vi "mtg reader - recolor folder list.vi"(6 "max index":i32, 9 "Row in":i32, 11 "table ref":refnum<vi>) -> (1 "Row out":i32, 3 "table ref out":refnum<vi>)   [LabVIEW 2025]
uses:
  <vilib>/Utility/miscctls.llb/LVRowAndColumnTypeDef.ctl
  <vilib>/Utility/miscctls.llb/LVRowAndColumnUnsignedTypeDef.ctl
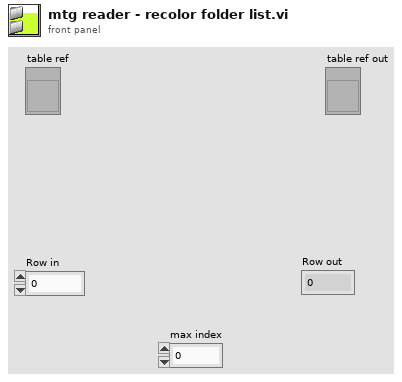
[diagram p1: front panel]
types:
  T1 = typedef "LVRowAndColumnUnsignedTypeDef.ctl" = cluster{"Row":u32, "Column":u32}
  T2 = typedef "LVRowAndColumnTypeDef.ctl" = cluster{"Row":i32, "Column":i32}
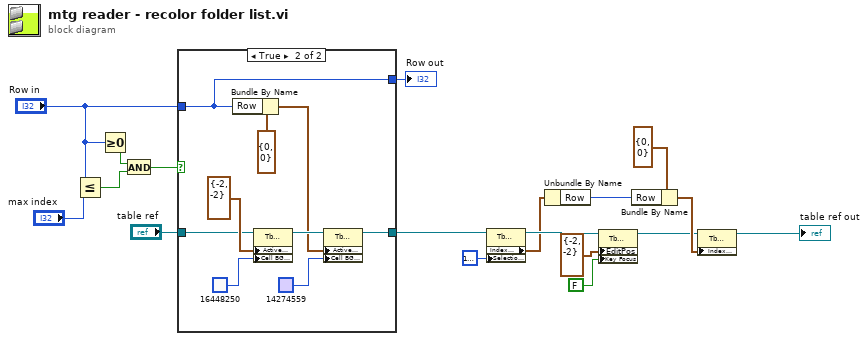
[diagram p0: block diagram]
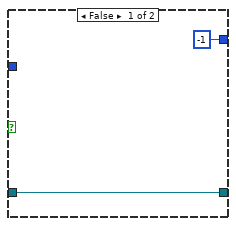
[diagram p2: hidden frame]
diagram:
  n1 = Less Or Equal?(x="Row in", y="max index") -> (x <= y?=w14:bool)
  n2 = Greater Or Equal To 0?(x="Row in") -> (x >= 0?=w15:bool)
  n3 = And(x=w15, y=w14) -> (x .and. y?=w13:bool)
  n4 = case shown="True" w13 {
    tunnel: "table ref" -> [w20 w24]
    tunnel: [w20 w22] -> w3
    tunnel: "Row in" -> [_ w21]
    tunnel: [-1 ("Row") w21] -> w12
    frame False {
    }
    frame True {
      n5 = Bundle By Name(cluster=T2 {"Row"=0, "Column"=0} ("Active Cell:Active Cell"), "Row"=w21) -> (w28:T2)
      n6 = property class="Tbl (strict)"(reference=w24, "Active Cell"=T2 {"Row"=-2, "Column"=-2} ("Active Cell:Active Cell"), "Cell BG Color"=u32 16448250 ("Active Cell:Cell Background Color")) -> (reference out=w29:refnum<vi>)  [unwired: 1 in, 1 out]
      n7 = property class="Tbl (strict)"(reference=w29, "Active Cell"=w28, "Cell BG Color"=u32 14274559 ("Active Cell:Cell Background Color")) -> (reference out=w22:refnum<vi>)  [unwired: 1 in, 1 out]
    }
  }
  "Row out" <- w12
  n8 = property class="Tbl (strict)"(reference=w3, "Selection Color"=u32 16777216) -> (reference out=w7:refnum<vi>, "Index Values"=w4:T1)  [unwired: 1 in, 1 out]
  n9 = Unbundle By Name(w4) -> ("Row"=w10:u32)
  n10 = property class="Tbl (strict)"(reference=w7, "EditPos"=T2 {"Row"=-2, "Column"=-2} ("Edit Position"), "Key Focus"=FALSE) -> (reference out=w8:refnum<vi>)  [unwired: 1 in, 1 out]
  n11 = Bundle By Name(cluster=T1 {"Row"=0, "Column"=0} ("Index Values"), "Row"=w10) -> (w11:T1)
  n12 = property class="Tbl (strict)"(reference=w8, "Index Values"=w11) -> (reference out=→"table ref out":refnum<vi>)  [unwired: 1 in, 1 out]
